vi "Check File Size.vi"(8 "error in (no error)":errorcluster, 11 "Text File in":refnum<class "Text File.lvclass">) -> (0 "error out":errorcluster, 3 "Text File out":refnum<class "Text File.lvclass">)   [LabVIEW 2019, in "TSC Event Logger.lvlib" / "Text File.lvclass"]
doc: "Check if the file size is beyond the maximum allowable for the text file sink.\n\n<b>Code Developed By:</b>\nTechnology Service Corporation\nBloomington, IN 47403\nwww.tsc.com/atcs\n\nDeveloper:\nDaniel Coons"
uses:
  Text File.lvclass
  Text File.lvclass/Text File.ctl
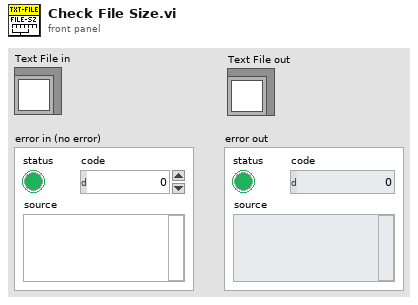
[diagram p1: front panel]
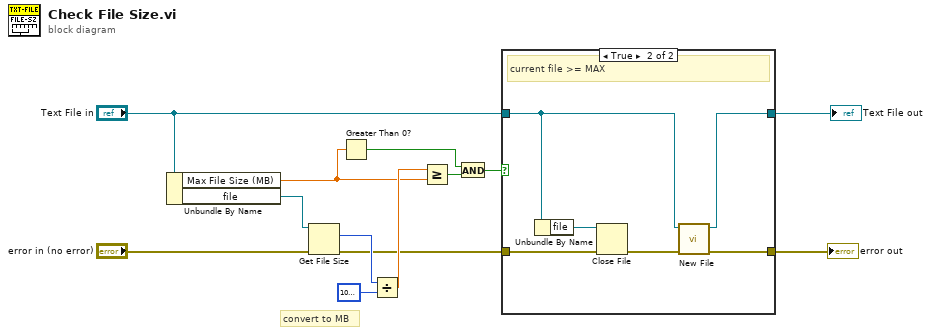
[diagram p0: block diagram]
diagram:
  # "convert to MB"
  n1 = Unbundle By Name("Text File in") -> ("Max File Size (MB)"=w3:dbl, "file"=w10:refnum<file>)
  n2 = Get File Size(file=w10, error in="error in (no error)") -> (size (in bytes)=w11:i64, 0:w8:errorcluster)  [unwired: 1 out]
  n3 = Greater Than 0?(x=w3) -> (x > 0?=w1:bool)
  n4 = Divide(x=w11, y=i64 1000000) -> (x/y=w13:dbl)
  n5 = Greater Or Equal?(x=w13, y=w3) -> (x >= y?=w4:bool)
  n6 = And(x=w1, y=w4) -> (x .and. y?=w2:bool)
  n7 = case shown="True" w2 {
    tunnel: w8 -> [w14 w16]
    tunnel: "Text File in" -> [w15 w19]
    tunnel: [w15 w20] -> w6
    tunnel: [w14 w21] -> w5
    frame False {
      # "file size fine, no change"
    }
    frame True {
      # "current file >= MAX"
      n8 = Unbundle By Name(w19) -> ("file"=w18:refnum<file>)
      n9 = Close File(refnum=w18, error in=w16) -> (error out=w17:errorcluster)  [unwired: 1 out]
      n10 = call "New File.vi"("Error In"=w17, "Text File in"=w19) -> ("error out"=w21:errorcluster, "Text File out"=w20:refnum<class "Text File.lvclass">)  [unwired: 8 in]
    }
  }
  "error out" <- w5
  "Text File out" <- w6
